vi "Gyro.vi"(0 "reset integrator":bool, 1 "[ESC]":bool) -> (6 "Linear Acceleration [LSB/sec^2]":cluster{i16, i16, i16}(graph), 7 "Z displacement":dbl format="%#_5g", 8 "X acc":i16, 9 "Y displacement":dbl format="%#_5g", 10 "Y acc":i16, 11 "X displacement":dbl format="%#_5g", 12 "Angular rate [LSB/sec]":cluster{dbl, dbl, dbl}(graph), 13 "Y rot rate":i16, 14 "Z acc":i16, 15 "Z rot rate":i16, 16 "Temp":i16, 17 "Angular displacement [LSB]":T2(graph), 18 "X rot rate":i16)   [LabVIEW 2017]
uses:
  <vilib>/myRIO/Instrument Drivers/Onboard IO/I2C/typedefs/I2C User Configuration.ctl
  <vilib>/myRIO/Instrument Drivers/Onboard IO/I2C/typedefs/I2C Transfer Rate.ctl
  <vilib>/Platform/TimedLoop/XDataNode/timing_clust.ctl
  <vilib>/Platform/TimedLoop/XDataNode/nitl_modes.ctl
  <vilib>/Platform/TimedLoop/XDataNode/wakeup.ctl
  <vilib>/myRIO/Common/Instrument Driver Framework/myRIO v1.0/DIO/vis/myRIO v1.1 Open DIO.vi
  <vilib>/myRIO/Common/Instrument Driver Framework/myRIO v1.0/I2C/vis/myRIO v1.1 Open I2C.vi
  <vilib>/myRIO/Common/Instrument Driver Framework/myRIO v1.0/UART/vis/myRIO v1.0 Close UART.vi
  <vilib>/myRIO/Common/Instrument Driver Framework/Utilities/vis/Validate Channels.vi
  <vilib>/myRIO/Common/Instrument Driver Framework/myRIO v1.0/DIO/vis/myRIO v1.0 Reserve DIO.vi
  <vilib>/myRIO/Common/Instrument Driver Framework/myRIO v1.0/I2C/vis/myRIO v1.0 Reserve I2C.vi
  <vilib>/myRIO/Common/Instrument Driver Framework/myRIO v1.0/Resource Manager/vis/myRIO v1.0 Reserve Channel List.vi
  <vilib>/myRIO/Common/Instrument Driver Framework/myRIO v1.0/DIO/vis/myRIO v1.0 Build MUX Configuration DIO.vi
  <vilib>/myRIO/Common/Instrument Driver Framework/myRIO v1.0/I2C/vis/myRIO v1.0 Build MUX Configuration I2C.vi
  <vilib>/myRIO/Common/Instrument Driver Framework/myRIO v1.0/Resource Manager/vis/myRIO v1.0 Reserve Channel.vi
  <vilib>/myRIO/Common/Instrument Driver Framework/myRIO v1.0/Resource Manager/vis/myRIO v1.0 Unreserve Channel.vi
  <vilib>/myRIO/Common/Instrument Driver Framework/myRIO v1.0/Resource Manager/vis/myRIO v1.0 Create Configuration List.vi
  <vilib>/myRIO/Common/Instrument Driver Framework/myRIO v1.0/Resource Manager/vis/myRIO v1.0 Build Mutex Name.vi
  <vilib>/Utility/VariantDataType/GetNumericInfo.vi
  <vilib>/Utility/error.llb/Error Cluster From Error Code.vi
  <vilib>/myRIO/Common/Instrument Driver Framework/myRIO v1.0/myRIO v1.1 Open.vi
  <vilib>/myRIO/Common/Instrument Driver Framework/Utilities/vis/IO Manager.vi
  <vilib>/myRIO/Common/Instrument Driver Framework/Utilities/vis/Configuration Manager.vi
  <vilib>/myRIO/Common/Instrument Driver Framework/myRIO v1.0/Resource Manager/vis/myRIO v1.0 Configure IO.vi
  <vilib>/myRIO/Common/Instrument Driver Framework/myRIO v1.0/myRIO v1.0 Close.vi
  <vilib>/myRIO/Common/Instrument Driver Framework/myRIO v1.0/I2C/vis/myRIO v1.0 Configure I2C.vi
  <vilib>/myRIO/Common/Instrument Driver Framework/myRIO v1.0/I2C/vis/myRIO v1.0 Write I2C.vi
  <vilib>/myRIO/Common/Instrument Driver Framework/myRIO v1.0/DIO/vis/myRIO v1.0 Read DIO.vi
  <vilib>/myRIO/Common/Instrument Driver Framework/myRIO v1.0/I2C/vis/myRIO v1.0 Read I2C.vi
  <vilib>/myRIO/Common/Instrument Driver Framework/Utilities/vis/FPGA Ref Manager.vi
  <vilib>/myRIO/Common/Instrument Driver Framework/myRIO v1.0/myRIO v1.0 Reset FPGA.vi
  <vilib>/myRIO/Common/Instrument Driver Framework/myRIO v1.0/IRQ/vis/myRIO v1.0 IRQ Info FGV.vi
  <vilib>/myRIO/Common/Instrument Driver Framework/myRIO v1.0/IRQ/vis/myRIO v1.0 Timer IRQ Info FGV.vi
  <vilib>/myRIO/Common/Instrument Driver Framework/myRIO v1.0/IRQ/vis/myRIO v1.0 ISR Agent.vi
  <vilib>/Platform/TimedLoop/XDataNode/XDataNode.xnode
  <vilib>/myRIO/Instrument Drivers/Utilities/Utilities.lvlib
  <vilib>/myRIO/Instrument Drivers/Onboard IO/I2C/I2C.lvlib
  <vilib>/myRIO/Instrument Drivers/Onboard IO/DIO/DIO.lvlib
  <vilib>/Platform/TimedLoop/XDataNode/XDNodeRunTimeDep.lvlib
  <vilib>/ptbypt/NI_PtbyPt.lvlib
panel:
  out "Waveform Chart":T1(graph)
  in  "Duty Cycle MCC2 : Faixa de operação":dbl(slide) scale=0.0..1.0
  in  "Controle sentido M2":bool
  in  "Duty Cycle MCC1 : Faixa de operação":dbl(slide) scale=0.0..1.0
  in  "Ligar (StandBy)":bool
  in  "Controle sentido M1":bool
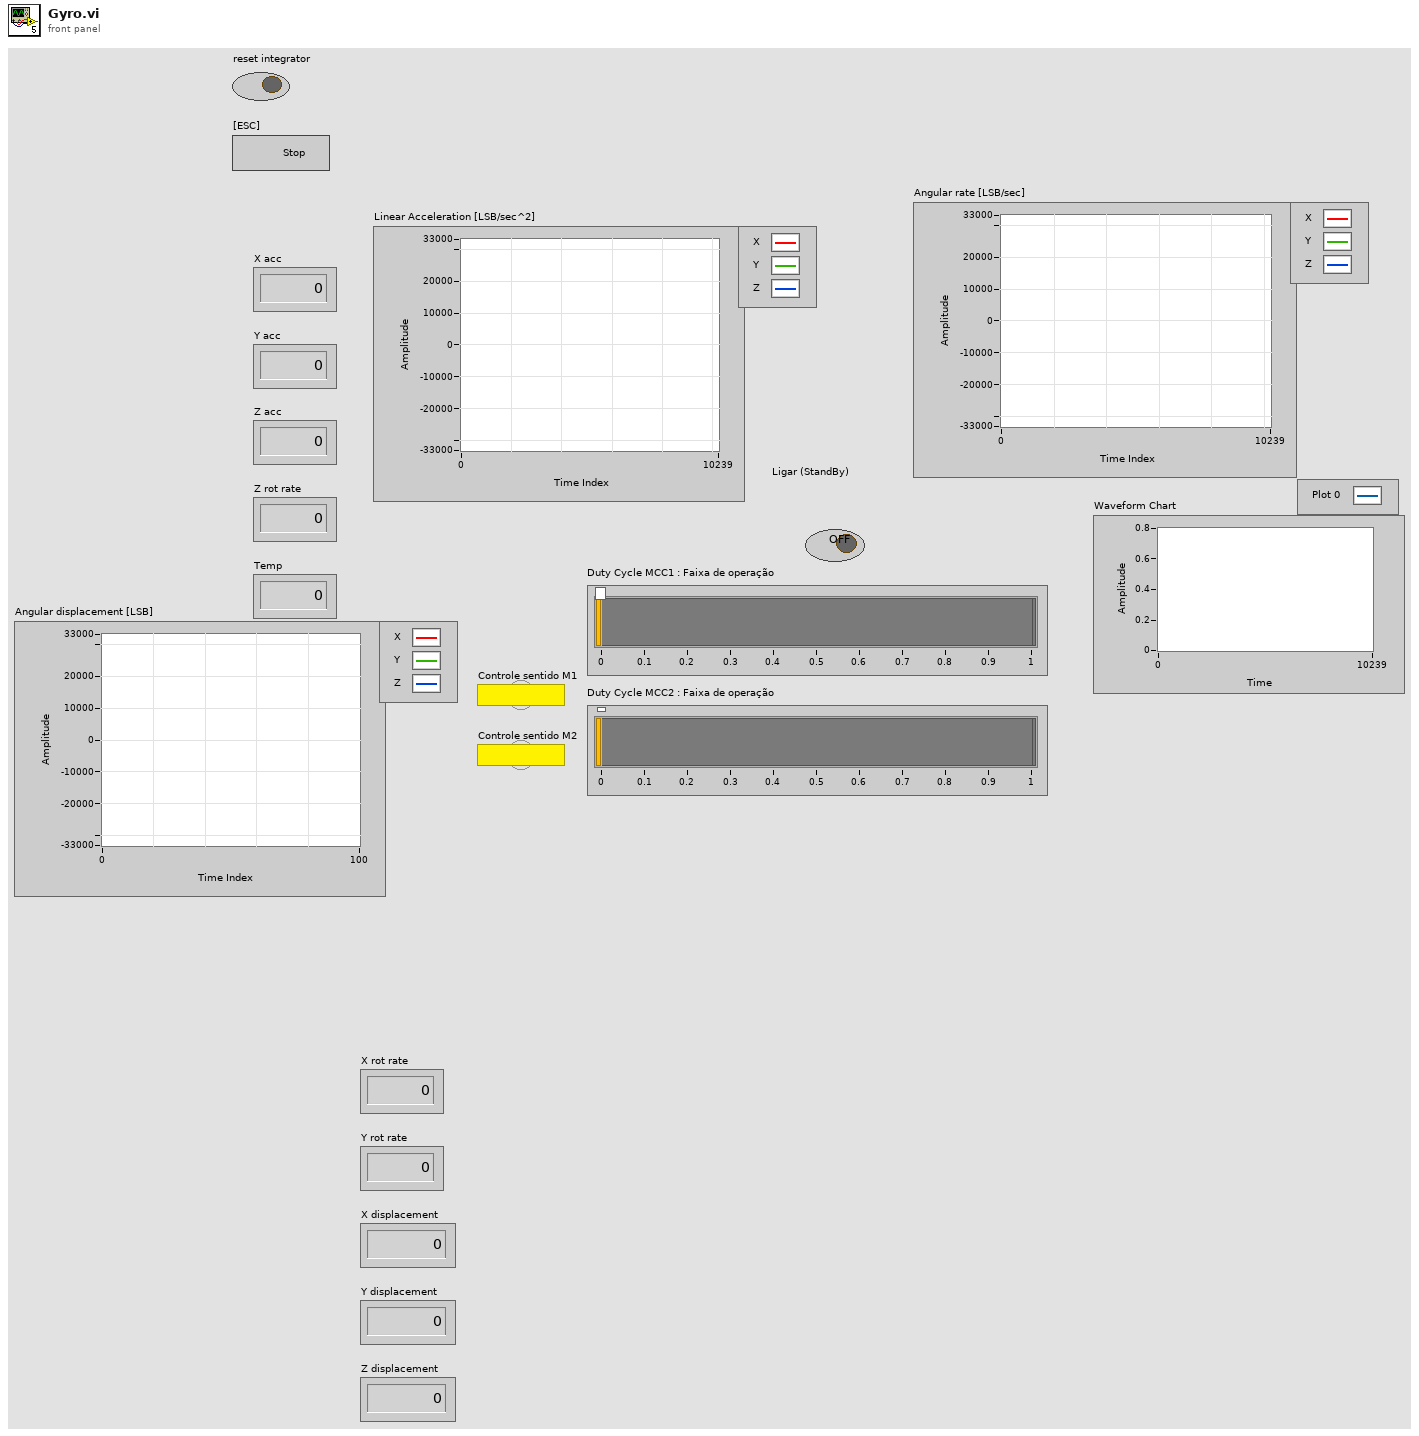
[diagram p1: front panel]
types:
  T1 = cluster{"\nDuty Cycle MCC2 : Faixa de operação  out":dbl, "\nDuty Cycle MCC1 : Faixa de operação out":dbl}
  T2 = cluster{"integral x(t)":dbl, "integral x(t)":dbl, "integral x(t)":dbl}
  T3 = typedef "I2C.lvlib/I2C User Configuration.ctl" = cluster{"I2C Transfer Rate":T4}
  T4 = typedef "I2C.lvlib/I2C Transfer Rate.ctl" = enum16{"Standard mode (100 kbps)", "Fast mode (400 kbps)"}
  T5 = typedef "I2C.lvlib/I2C Reference.ctl" = cluster{"myRIO Reference":T6, "I2C Channels Enum":T10, "I2C Configuration":T11}
  T6 = typedef "myRIO Generic Hardware Reference.ctl" = cluster{"myRIO Model":T7, "myRIO Hardware Reference":T8}
  T7 = typedef "Hardware Version Enum.ctl" = enum16{"Unknown", "myRIO-1900", "myRIO-1950", "roboRIO", "NI ELVIS RIO CM"}
  T8 = typedef "myRIO v1.0 Reference.ctl" = cluster{"Generic FPGA Reference":T9, "Allow multiple opens":bool}
  T9 = typedef "Generic FPGA Reference.ctl" = refnum<k20>
  T10 = typedef "I2C Channels Enum.ctl" = enum16{"Not Connected", "A/I2C", "B/I2C", "I2C/I2C"}
  T11 = typedef "I2C.lvlib/I2C Configuration.ctl" = cluster{"I2C Transfer Rate":T4}
  T12 = typedef "DIO.lvlib/DIO Reference.ctl" = cluster{"myRIO Reference":T6, "DIO Channels List":T13}
  T13 = typedef "DIO Channels List.ctl" = T14[]
  T14 = typedef "DIO Channels Enum.ctl" = enum16{"Not Connected", "C/DIO0", "C/DIO1", "C/DIO2", "C/DIO3", "C/DIO4", "C/DIO5", "C/DIO6", "C/DIO7", "A/DIO0", "A/DIO1", "A/DIO2", "A/DIO3", "A/DIO4", "A/DIO5", "A/DIO6", "A/DIO7", "A/DIO8", "A/DIO9", "A/DIO10", "A/DIO11", "A/DIO12", "A/DIO13", "A/DIO14", "A/DIO15", "B/DIO0", "B/DIO1", "B/DIO2", "B/DIO3", "B/DIO4", "B/DIO5", "B/DIO6", "B/DIO7", "B/DIO8", "B/DIO9", "B/DIO10", "B/DIO11", "B/DIO12", "B/DIO13", "B/DIO14", "B/DIO15", "LED0", "LED1", "LED2", "LED3", "Button0", "DIO/DIO0", "DIO/DIO1", "DIO/DIO2", "DIO/DIO3", "DIO/DIO4", "DIO/DIO5", "DIO/DIO6", "DIO/DIO7", "DIO/DIO8", "DIO/DIO9", "SPI/CS0", "SPI/CS1", "SPI/CS2", "SPI/CS3", "LED RADIO (Green)", "LED RADIO (Red)", "LED COMM (Green)", "LED COMM (Red)", "LED MODE (Green)", "LED MODE (Red)"}
  T15 = typedef "XDNodeRunTimeDep.lvlib/timing_clust.ctl" = cluster{"Expected End [f-1]":u64, "Actual End [f-1]":u64, "Finished Late? [f-1]":bool, "Expected End [i-1]":u64, "Actual End [i-1]":u64, "Finished Late? [i-1]":bool, "Expected Start [i]":u64, "Actual Start [i]":u64, "Expected Start [f]":u64, "Actual Start [f]":u64, "Source Name":string, "Structure Name":string, "Period":i64, "Deadline":i64, "Offset":i64, "Start":i64, "Priority":i32, "Timeout":i32, "Mode":T16, "Wakeup Reason":T17, "Error":errorcluster, "Source Type":string, "Secondary Source Type":string, "Global End Time":u64, "Global Start Time":u64, "Frame Duration":u64, "Iteration Duration":u64, "Assigned CPU":i32, "I/O Scan Engine Mode":u32}
  T16 = typedef "XDNodeRunTimeDep.lvlib/nitl_modes.ctl" = enum32{"No Change", "Process missed periods, maintain original phase", "Discard missed periods, maintain original phase", "Process missed periods, ignore original phase", "Discard missed periods, ignore original phase"}
  T17 = typedef "XDNodeRunTimeDep.lvlib/wakeup.ctl" = enum32{"Normal", "Aborted", "Asynchronous wakeup", "Timing source error", "Timed loop error", "Timeout"}
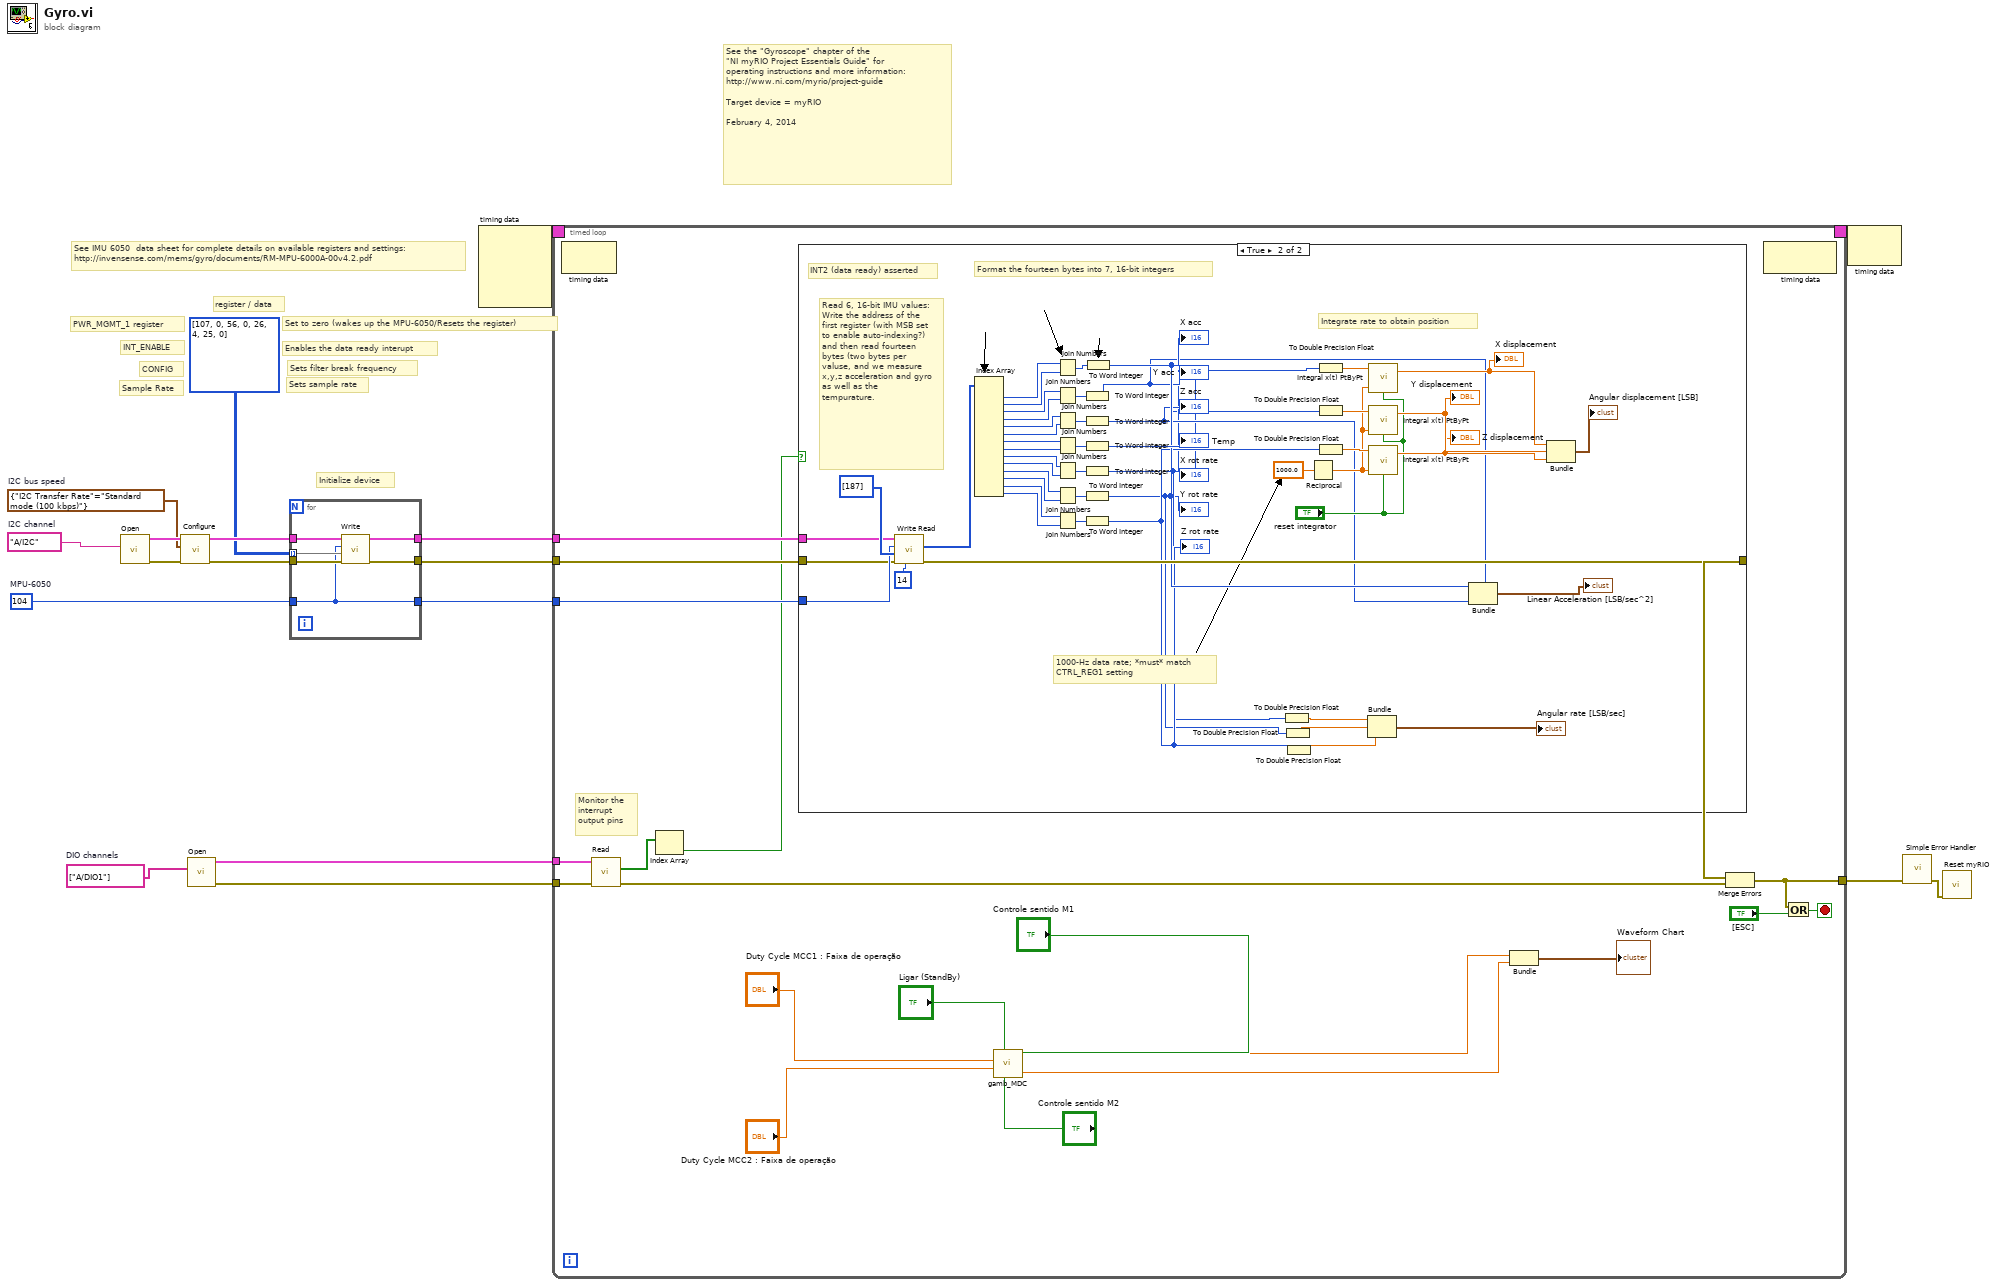
[diagram p0: block diagram]
diagram:
  w14 = tag[] ["A/DIO1"]  # DIO channels
  w3 = T3 {"I2C Transfer Rate"=enum."Standard mode (100 kbps)"}  # I2C bus speed
  w16 = tag "A/I2C"  # I2C channel
  w12 = u8 104  # MPU-6050
  # "Sets sample rate"
  # "Sample Rate"
  # "Sets filter break frequency"
  # "CONFIG"
  # "INT_ENABLE"
  # "Enables the data ready interupt"
  # "See the \"Gyroscope\" chapter of the\n\"NI myRIO Project Essentials Guide\" for\noperating instructions and more information: \nhttp://www.ni.com/myrio/project-guide\n\nTarget device = myRIO\n\nFebruary 4, 2014"
  # "Set to zero (wakes up the MPU-6050/Resets the register)"
  # "PWR_MGMT_1 register"
  # "Initialize device"
  # "See IMU 6050  data sheet for complete details on available registers and settings:\nhttp://invensense.com/mems/gyro/documents/RM-MPU-6000A-00v4.2.pdf"
  # "register / data"
  n1 = call <vilib>:"Open.vi"("Channel Name"=w16) -> ("error out"=w5:errorcluster, "I2C Ref Out"=w4:T5)  [unwired: 9 in]
  n2 = call <vilib>:"Configure.vi"("error in (no error)"=w5, "I2C User Configuration"=w3, "I2C Ref In"=w4) -> ("error out"=w11:errorcluster, "I2C Ref Out"=w10:T5)  [unwired: 7 in]
  n3 = call <vilib>:"Open.vi"("Channel Names"=w14) -> ("error out"=w13:errorcluster, "DIO Ref Out"=w15:T12)  [unwired: 9 in]
  n4 = for {
    tunnel: [w24] -> w6
    tunnel: [w23] -> w7
    tunnel: [w19] -> w8
    tunnel: u8[][] [[107, 0], [56, 0], [26, 4], [25, 0]] ("Bytes to Write") -> [w22] mode=indexing
    tunnel: w10 -> [w21]
    tunnel: w11 -> [w20]
    tunnel: w12 -> [w19]
    n5 = call <vilib>:"Write.vi"("error in (no error)"=w20, "Bytes to Write"=w22, "Slave Address (7-bit)"=w19, "I2C Ref In"=w21) -> ("error out"=w24:errorcluster, "I2C Ref Out"=w23:T5)  [unwired: 6 in]
  }
  n6 = node-c288() -> (w18:T15)  [unwired: 4 in]
  n7 = timed-loop {
    tunnel: [w35] -> w2
    tunnel: w8 -> [w40]
    tunnel: w6 -> [w42]
    tunnel: w7 -> [w41]
    tunnel: w13 -> [w39]
    timing: w18 -> [_]
    timing-out: [_] -> w17
    tunnel: w15 -> [w34]
    stop <- w44 stop-if-true
    # "Monitor the\ninterrupt\noutput pins"
    n8 = node-c288() -> ()  [unwired: 1 in, 1 out]
    n9 = call <vilib>:"Read.vi"("error in (no error)"=w39, "DIO Ref In"=w34) -> ("error out"=w33:errorcluster, "Values"=w36:bool[])  [unwired: 7 in, 1 out]
    n10 = Index Array "Index Array"(array=w36) -> (element=w37:bool)  [unwired: 1 in]
    n11 = case shown="True" w37 {
      tunnel: w42 -> [w47 w85]
      tunnel: w41 -> [_ w86]
      tunnel: w40 -> [_ w92]
      tunnel: [w47 w91] -> w38
      frame False {
        # "INT2 (data ready) deasserted"
      }
      frame True {
        # "1000-Hz data rate; *must* match\nCTRL_REG1 setting"
        # "Integrate rate to obtain position"
        # "INT2 (data ready) asserted"
        # "Read 6, 16-bit IMU values:\nWrite the address of the first register (with MSB set to enable auto-indexing?) and then read fourteen bytes (two bytes per valuse, and we measure x,y,z acceleration and gyro as well as the tempurature."
        # "Format the fourteen bytes into 7, 16-bit integers"
        n12 = call <vilib>:"Write Read.vi"("Byte Count"=u32 14, "error in (no error)"=w85, "Bytes to Write"=u8[] [187], "Slave Address (7-bit)"=w92, "I2C Ref In"=w86) -> ("error out"=w91:errorcluster, "Bytes Read"=w90:u8[])  [unwired: 3 in, 1 out]
        n13 = Index Array "Index Array"(array=w90) -> (element #1=w77:u8, element #2=w76:u8, element #3=w75:u8, element #4=w74:u8, element #5=w73:u8, element #6=w72:u8, element #7=w71:u8, element #8=w70:u8, element #9=w69:u8, element #10=w68:u8, element #11=w67:u8, element #12=w66:u8, element #13=w65:u8, element #14=w64:u8)  [unwired: 14 in]
        n14 = Join Numbers(hi=w77, lo=w76) -> ((hi.lo)=w97:u16)
        n15 = Join Numbers(hi=w75, lo=w74) -> ((hi.lo)=w96:u16)
        n16 = Join Numbers(hi=w73, lo=w72) -> ((hi.lo)=w95:u16)
        n17 = Join Numbers(hi=w71, lo=w70) -> ((hi.lo)=w63:u16)
        n18 = Join Numbers(hi=w69, lo=w68) -> ((hi.lo)=w62:u16)
        n19 = Join Numbers(hi=w67, lo=w66) -> ((hi.lo)=w61:u16)
        n20 = Join Numbers(hi=w65, lo=w64) -> ((hi.lo)=w60:u16)
        n21 = To Word Integer(number=w96) -> (16bit integer=w55:i16)
        "Y acc" <- w55
        n22 = To Word Integer(number=w95) -> (16bit integer=w54:i16)
        "Z acc" <- w54
        n23 = To Word Integer(number=w63) -> (16bit integer=→"Temp":i16)
        n24 = To Word Integer(number=w62) -> (16bit integer=w51:i16)
        "X rot rate" <- w51
        n25 = To Word Integer(number=w61) -> (16bit integer=w49:i16)
        "Y rot rate" <- w49
        n26 = To Word Integer(number=w60) -> (16bit integer=w53:i16)
        "Z rot rate" <- w53
        n27 = To Word Integer(number=w97) -> (16bit integer=w56:i16)
        "X acc" <- w56
        n28 = To Double Precision Float(number=w51) -> (double precision float=w50:dbl)
        n29 = To Double Precision Float(number=w49) -> (double precision float=w48:dbl)
        n30 = To Double Precision Float(number=w53) -> (double precision float=w52:dbl)
        n31 = Reciprocal(x=1000.0 ("dt")) -> (1/x=w83:dbl)
        n32 = To Double Precision Float(number=w51) -> (double precision float=w78:dbl)
        n33 = To Double Precision Float(number=w49) -> (double precision float=w89:dbl)
        n34 = To Double Precision Float(number=w53) -> (double precision float=w88:dbl)
        n35 = Bundle "Bundle"(w50, w48, w52) -> (→"Angular rate [LSB/sec]":cluster{dbl, dbl, dbl})  [unwired: 1 in]
        n36 = call <vilib>:"Integral x(t) PtByPt.vi"("initialize"="reset integrator", "dt"=w83, "x"=w78) -> ("integral x(t)"=w79:dbl)  [unwired: 1 in, 1 out]
        "X displacement" <- w79
        n37 = call <vilib>:"Integral x(t) PtByPt.vi"("initialize"="reset integrator", "dt"=w83, "x"=w89) -> ("integral x(t)"=w82:dbl)  [unwired: 1 in, 1 out]
        "Y displacement" <- w82
        n38 = call <vilib>:"Integral x(t) PtByPt.vi"("initialize"="reset integrator", "dt"=w83, "x"=w88) -> ("integral x(t)"=w81:dbl)  [unwired: 1 in, 1 out]
        "Z displacement" <- w81
        n39 = Bundle "Bundle"(w56, w55, w54) -> (→"Linear Acceleration [LSB/sec^2]":cluster{i16, i16, i16})  [unwired: 1 in]
        n40 = Bundle "Bundle"("integral x(t)"=w79, "integral x(t)"=w82, "integral x(t)"=w81) -> (→"Angular displacement [LSB]":T2)  [unwired: 1 in]
      }
    }
    n41 = call "gamb_MDC.vi"("Controle sentido M2"="Controle sentido M2", "Ligar (StandBy)"="Ligar (StandBy)", "Duty Cycle MCC2 : Faixa de operação  in"="Duty Cycle MCC2 : Faixa de operação", "Duty Cycle MCC1 : Faixa de operação in"="Duty Cycle MCC1 : Faixa de operação", "Controle sentido M1"="Controle sentido M1") -> ("Duty Cycle MCC1 : Faixa de operação out"=w26:dbl, "Duty Cycle MCC2 : Faixa de operação  out"=w27:dbl)  [unwired: 5 in]
    n42 = Bundle "Bundle"("Duty Cycle MCC2 : Faixa de operação  out"=w27, "Duty Cycle MCC1 : Faixa de operação out"=w26) -> (→"Waveform Chart":T1)  [unwired: 1 in]
    n43 = Merge Errors "Merge Errors"(w38, w33) -> (w35:errorcluster)
    n44 = node-c288() -> ()  [unwired: 1 in, 1 out]
    n45 = Or(x=w35, y="[ESC]") -> (x .or. y?=w44:bool)
  }
  n46 = node-c288(w17) -> ()  [unwired: 1 out]
  n47 = call <vilib>:"Simple Error Handler.vi"("error in (no error)"=w2) -> ("error out"=w1:errorcluster)  [unwired: 4 in, 4 out]
  n48 = call <vilib>:"Reset myRIO.vi"("error in (no error)"=w1) -> ()  [unwired: 10 in, 1 out]
